vi "Data FGV.vi"(7 "Write?":bool=TRUE, 11 "Data In":T1 {"Time" format="%<%H:%M:%S%2u>T"}) -> (3 "Data Out":T1 {"Time" format="%<%H:%M:%S%2u>T"})   [LabVIEW 2015]
uses:
  Global Data.ctl
  Data.ctl
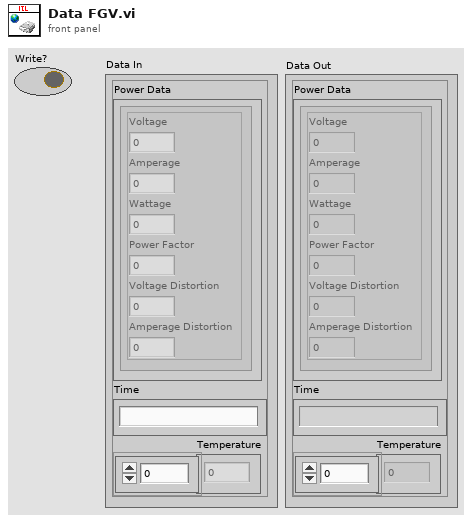
[diagram p1: front panel]
types:
  T1 = typedef "Global Data.ctl" = cluster{"Power Data":T2[], "Time":timestamp, "Temperature":dbl[]}
  T2 = typedef "Data.ctl" = cluster{"Voltage":dbl, "Amperage":dbl, "Wattage":dbl, "Power Factor":dbl, "Voltage Distortion":dbl, "Amperage Distortion":dbl}
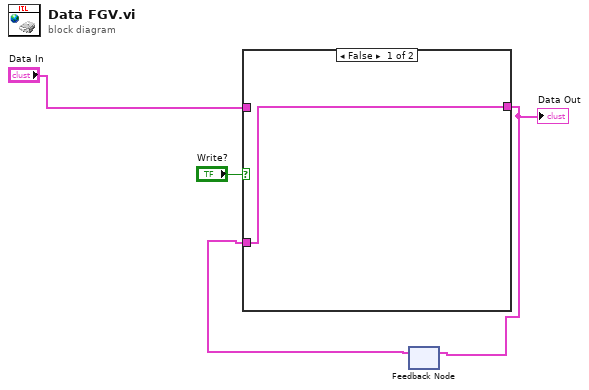
[diagram p0: block diagram]
diagram:
  n1 = feedback #1() -> (w3:T1)  [unwired: 1 in]
  n2 = case shown="False" "Write?" {
    tunnel: "Data In" -> [_ w6]
    tunnel: [w5 w6] -> w2
    tunnel: w3 -> [w5 _]
    frame False {
    }
    frame True {
    }
  }
  "Data Out" <- w2
  n3 = feedback-in #1(w2) -> ()
